vi "Configure Edge Trigger Source Core.vi"(0 "CS++Scope":refnum<class "CS++Scope.lvclass">, 5 "trigger source (CHANNEL1)":string(combo)="CHANNEL1" caption="trigger source (\"CHANNEL1\")", 7 "trigger slope (Positive)":i32(ring)=1 items=["Positive"=1, "Negative"=0], 9 "trigger level  (0.0 V)":dbl[unit] format="%.3f", 11 "error in (no error)":errorcluster) -> (4 "CS++Scope out":refnum<class "CS++Scope.lvclass">, 15 "error out":errorcluster)   [LabVIEW 2015, in "CS++Scope.lvlib" / "CS++Scope.lvclass"]
doc: "This VI configures the edge trigger. An edge trigger occurs when the trigger signal passes through the voltage threshold that you specify with the Trigger Level parameter and has the slope that you specify with the Trigger Slope parameter. \n\nNotes:\n (1) This VI affects instrument behavior only if the trigger type is\n IVISCOPE_VAL_EDGE_TRIGGER. Call the IviScope Configure Trigger and\n IviScope Configure Trigger Coupling VIs to set the trigger type and trigger coupling\n before calling this VI.\n (2) If the trigger source is one of the analog input channels, you must configure\n the vertical range, vertical offset, vertical coupling, probe attenuation, and the\n maximum input frequency before calling this VI."
uses:
  CS++Scope.lvclass
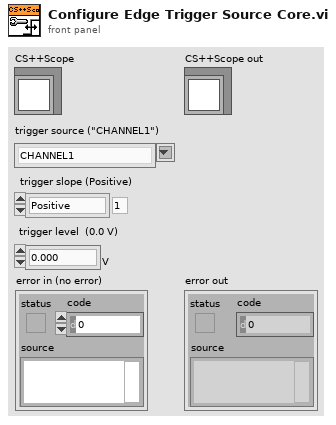
[diagram p1: front panel]
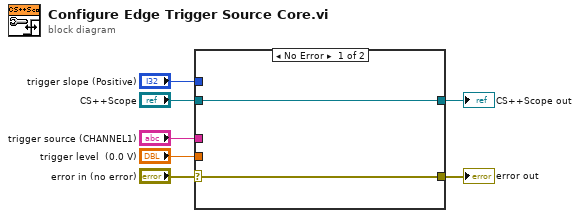
[diagram p0: block diagram]
diagram:
  n1 = case shown="No Error" "error in (no error)" {
    selector: "error in (no error)" -> [w8 w11]
    tunnel: [w8 w11] -> w6
    tunnel: [w9 w10] -> w2
    tunnel: "CS++Scope" -> [w9 w10]
    tunnel: "trigger source (CHANNEL1)" -> [_ _]
    tunnel: "trigger level  (0.0 V)" -> [_ _]
    tunnel: "trigger slope (Positive)" -> [_ _]
    frame No Error {
    }
    frame Error {
    }
  }
  "error out" <- w6
  "CS++Scope out" <- w2
